vi "L32.vi"() -> ()   [LabVIEW 2014]
panel:
  in  "L32":dbl
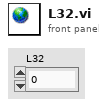
[diagram p1: front panel]
diagram:
